vi "Action Update Heater State-test-Caraya.vi"(8 "error in (no error)":errorcluster) -> (0 "error out":errorcluster)   [LabVIEW 2018]
uses:
  Libraries/Thermal Chamber Controller_DQMH/Heater State--enum.ctl
  <vilib>/addons/_JKI Toolkits/Caraya/classes/Assert/Assert True.vi
  <vilib>/addons/_JKI Toolkits/Caraya/classes/Test/Test.lvclass
  Libraries/Thermal Chamber Controller_DQMH/Thermal Chamber Controller_DQMH.lvlib
  <vilib>/addons/_JKI Toolkits/Caraya/classes/Assert/Assert.lvclass
  Libraries/Thermal Chamber Response Simulator/Thermal Chamber Response Simulator.lvlib
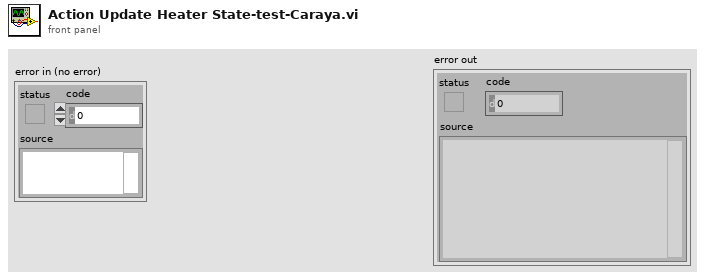
[diagram p1: front panel]
types:
  T1 = typedef "Thermal Chamber Controller_DQMH.lvlib/Heater State--enum.ctl" = enum16{"Heater Enabled", "Heater Disabled"}
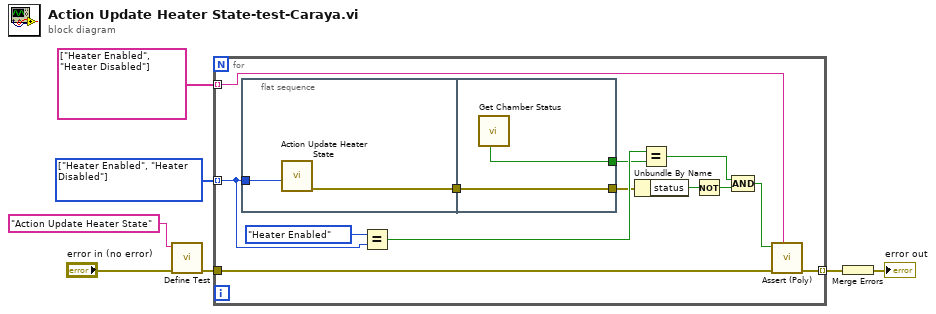
[diagram p0: block diagram]
diagram:
  w2 = T1[] [enum."Heater Enabled", enum."Heater Disabled"] items=["Heater Enabled", "Heater Disabled"] ("Array")
  n1 = call <vilib>:"Define Test.vi"("error in (no error)"="error in (no error)", "Label (VI Title)"="Action Update Heater State") -> ("error out"=w5:errorcluster)  [unwired: 9 in]
  n2 = for {
    tunnel: w5 -> [w20]
    tunnel: [w19] -> w3 mode=indexing
    tunnel: w2 -> [w12] mode=indexing
    tunnel: string[] ["Heater Enabled", "Heater Disabled"] -> [w8] mode=indexing
    n3 = flat-sequence {
      tunnel: w12 -> [w22]
      tunnel: [w21] -> w10
      tunnel: [w24] -> w11
      tunnel: w10 -> [w24]
      tunnel: [w23] -> w9
      frame #0 {
        n4 = call "Action Update Heater State.vi"("Heater State"=w22) -> ("error out"=w21:errorcluster)  [unwired: 10 in]
      }
      frame #1 {
        n5 = call "Get Chamber Status.vi"() -> ("Heater State"=w23:bool)  [unwired: 6 in, 5 out]
      }
    }
    n6 = Equal?(x=Heater_State--enum."Heater Enabled" ("Heater State Result"), y=w12) -> (x = y?=w14:bool)
    n7 = Unbundle By Name(w11) -> ("status"=w18:bool)
    n8 = Equal?(x=w14, y=w9) -> (x = y?=w17:bool)
    n9 = Not(x=w18) -> (.not. x?=w16:bool)
    n10 = Compound Arithmetic op=AND(w17, w16) -> (w13:bool)
    n11 = call-poly <vilib>:"Assert (Poly).vi"("Label"=w8, "error in (no error)"=w20, "True?"=w13) -> ("error out"=w19:errorcluster)  [unwired: 8 in]
  }
  n12 = Merge Errors(w3) -> (→"error out":errorcluster)
